vi "Galvo-Control-V1.vi"() -> ()   [LabVIEW 2024]
uses:
  <vilib>/Utility/error.llb/DialogType.ctl
  <vilib>/DAQmx/write.llb/DAQmx Write (Analog 2D DBL NChan NSamp).vi
  <vilib>/DAQmx/create/channels.llb/DAQmx Create Channel (AO-Voltage-Basic).vi
  <vilib>/DAQmx/configure/timing.llb/DAQmx Timing (Sample Clock).vi
  <vilib>/DAQmx/miscellaneous.llb/DAQmx Fill In Error Info.vi
  <vilib>/measure/NI_MABase.lvlib
panel:
  out "Y axis chart":dbl[](graph)
  out "X axis chart":dbl[](graph)
  in  "Y frequency":dbl=10.0 format="%0.2p"
  in  "amplitude (both)":dbl=1.0 format="%0.2p"
  in  "X frequency":dbl=10.0 format="%0.2p"
  in  "Offset (both)":dbl format="%0.2p"
  in  "Y axis channel":tag
  in  "stop":bool
  in  "X axis channel":tag
  # "cDAQ1Mod1/ao1"
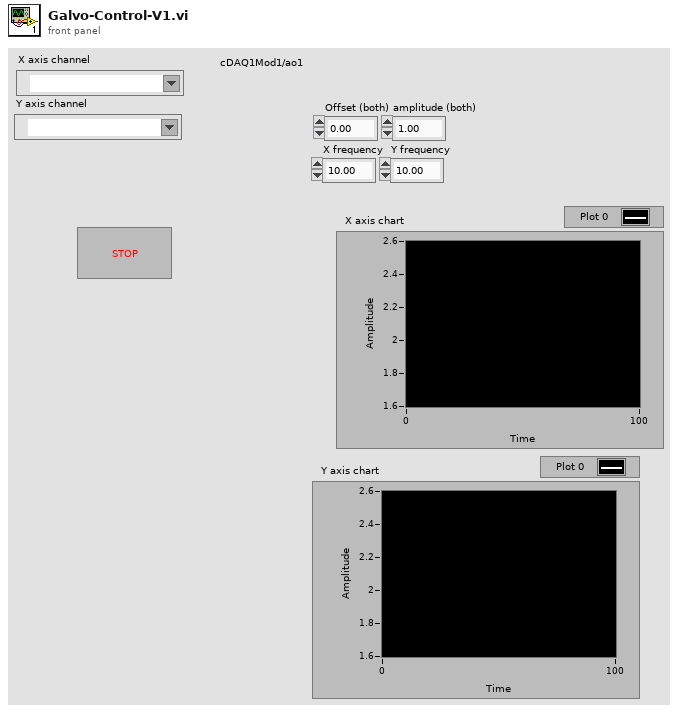
[diagram p1: front panel]
types:
  T1 = typedef "DialogType.ctl" = u16
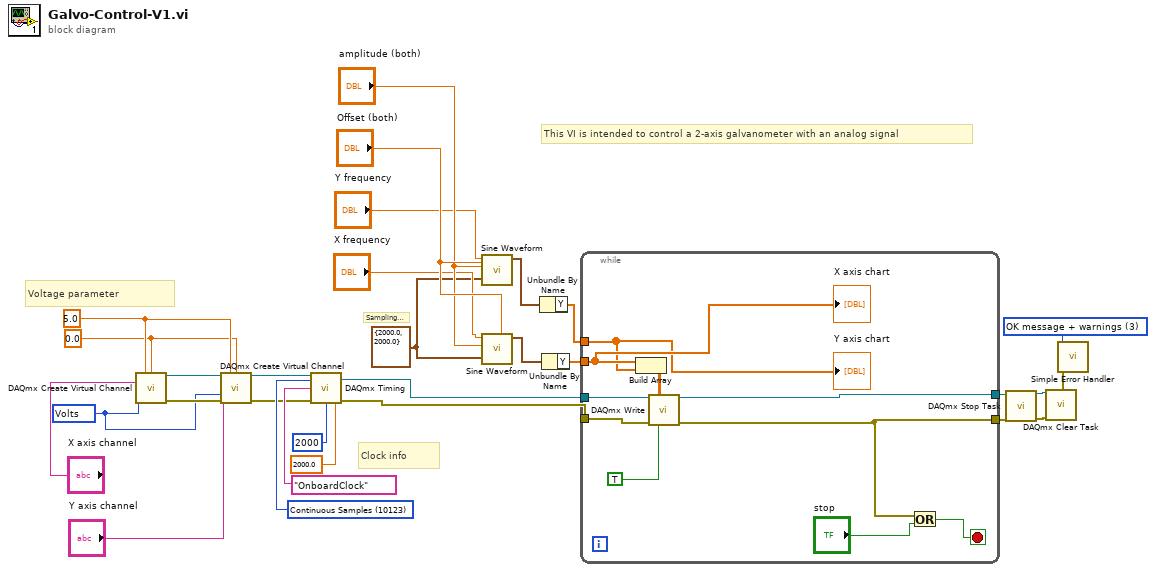
[diagram p0: block diagram]
diagram:
  w1 = cluster{"Fs":dbl, "#s":dbl} {"Fs"=2000.0, "#s"=2000.0} ("sampling info")
  w24 = 10123 items=["Finite Samples"=10178, "Continuous Samples"=10123, "Hardware Timed Single Point"=12522] ("sample mode")
  w10 = 10348 items=["Volts"=10348, "From Custom Scale"=10065] ("units")
  w11 = 0.0 ("minimum value")
  w12 = 5.0 ("maximum value")
  w27 = T1 3 items=["no dialog", "OK message", "continue or stop message", "OK message + warnings", "continue/stop + warnings"] ("type of dialog (OK msg:1)")
  # "This VI is intended to control a 2-axis galvanometer with an analog signal"
  # "Voltage parameter"
  # "Clock info"
  # "Sampling info"
  n1 = call-poly <vilib>:"DAQmx Create Virtual Channel.vi"("maximum value"=w12, "minimum value"=w11, "physical channels"="X axis channel", "units"=w10) -> ("task out"=w17:refnum<k21>, "error out"=w16:errorcluster)  [unwired: 10 in]
  n2 = call-poly <vilib>:"DAQmx Create Virtual Channel.vi"("task in"=w17, "maximum value"=w12, "minimum value"=w11, "physical channels"="Y axis channel", "units"=w10, "error in"=w16) -> ("task out"=w15:refnum<k21>, "error out"=w14:errorcluster)  [unwired: 8 in]
  n3 = call-poly <vilib>:"DAQmx Timing.vi"("task/channels in"=w15, "sample mode"=w24, "samples per channel"=2000, "rate"=2000.0, "source"=tag "OnboardClock", "error in"=w14) -> ("task out"=w20:refnum<k21>, "error out"=w19:errorcluster)  [unwired: 8 in]
  n4 = call <vilib>:"Sine Waveform.vi"("offset"="Offset (both)", "sampling info"=w1, "amplitude"="amplitude (both)", "frequency"="Y frequency") -> ("signal out"=w8:waveform(dbl))  [unwired: 6 in, 1 out]
  n5 = call <vilib>:"Sine Waveform.vi"("offset"="Offset (both)", "sampling info"=w1, "amplitude"="amplitude (both)", "frequency"="X frequency") -> ("signal out"=w9:waveform(dbl))  [unwired: 6 in, 1 out]
  n6 = Unbundle By Name(w8) -> ("Y"=w2:dbl[])
  n7 = Unbundle By Name(w9) -> ("Y"=w3:dbl[])
  n8 = while {
    tunnel: w20 -> [w38]
    tunnel: w19 -> [w37]
    tunnel: [w36] -> w23
    tunnel: [w35] -> w22
    tunnel: w3 -> [w32]
    tunnel: w2 -> [w31]
    stop <- w40 stop-if-true
    n9 = Build Array(w32, w31) -> (w33:dbl[][])
    n10 = call-poly <vilib>:"DAQmx Write.vi"("task/channels in"=w38, "auto start"=TRUE, "data"=w33, "error in"=w37) -> ("task out"=w36:refnum<k21>, "error out"=w35:errorcluster)  [unwired: 9 in, 1 out]
    n11 = Or(x=w35, y="stop") -> (x .or. y?=w40:bool)
    "X axis chart" <- w32
    "Y axis chart" <- w31
  }
  n12 = call <vilib>:"DAQmx Stop Task.vi"("task/channels in"=w23, "error in"=w22) -> ("task out"=w30:refnum<k21>, "error out"=w29:errorcluster)  [unwired: 12 in]
  n13 = call <vilib>:"DAQmx Clear Task.vi"("task in"=w30, "error in"=w29) -> ("error out"=w28:errorcluster)  [unwired: 13 in]
  n14 = call <vilib>:"Simple Error Handler.vi"("type of dialog (OK msg:1)"=w27, "error in (no error)"=w28) -> ()  [unwired: 3 in, 5 out]
